vi "Approve.vi"(8 "error in (no error)":errorcluster, 10 "Approver ID":i64, 11 "Submission in":refnum<class "Submission.lvclass">) -> (0 "error out":errorcluster, 3 "Submission out":refnum<class "Submission.lvclass">)   [LabVIEW 2020, in "Summer of LabVIEW.lvlib" / "Submission.lvclass"]
uses:
  Submission.lvclass
  Submission.lvclass/Submission.ctl
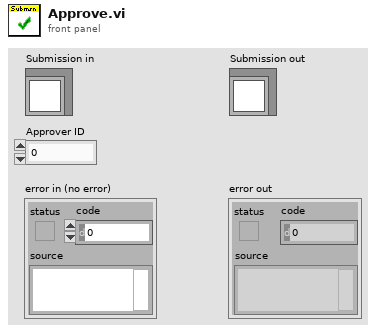
[diagram p1: front panel]
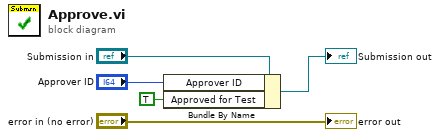
[diagram p0: block diagram]
diagram:
  n1 = Bundle By Name(cluster="Submission in", "Approver ID"="Approver ID", "Approved for Test"=TRUE ("Submission Data.Approved for Test")) -> (→"Submission out":refnum<class "Submission.lvclass">)
  "error out" <- "error in (no error)"
